vi "Launch Endpoint Actor.vi"(8 "error in (no error)":errorcluster, 11 "Test in":refnum<class "Test.lvclass">) -> (0 "error out":errorcluster, 3 "Test out":refnum<class "Test.lvclass">)   [LabVIEW 2019, in "Test.lvlib" / "Test.lvclass"]
uses:
  Test.lvclass
  C:/Program Files (x86)/National Instruments/LabVIEW 2019/vi.lib/ActorFramework/Actor/Actor.lvclass
  <vilib>/NI/Actors/Network Endpoint Actors/Nested Endpoint/Nested Endpoint/Nested Endpoint.lvclass
  C:/Program Files (x86)/National Instruments/LabVIEW 2019/vi.lib/NI/Actors/Network Endpoint Actors/Network Endpoint/Network Endpoint/Network Endpoint.lvclass
  Test Messages/Endpoint Connected Msg/Endpoint Connected Msg.lvclass
  C:/Program Files (x86)/National Instruments/LabVIEW 2019/vi.lib/NI/Actors/Network Endpoint Actors/Nested Endpoint/Nested Endpoint Messages/Connected Msg/Connected Msg.lvclass
  Test.lvclass/Test.ctl
  <vilib>/NI/Actors/Network Endpoint Actors/Network Endpoint/Network Endpoint/Network Endpoint.lvclass/Network Endpoint.ctl
  <vilib>/NI/Actors/Network Endpoint Actors/Nested Endpoint/Nested Endpoint/Nested Endpoint.lvclass/Nested Endpoint.ctl
  <vilib>/NI/Actors/Network Endpoint Actors/Network Endpoint/Network Endpoint/Network Endpoint.lvclass
  <vilib>/ActorFramework/Actor/Actor.lvclass
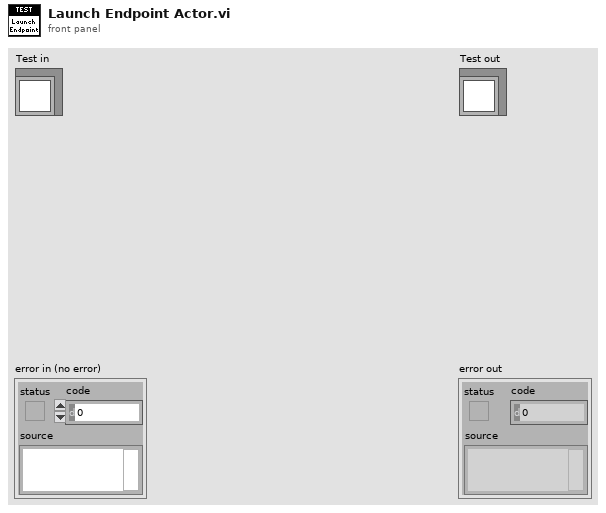
[diagram p1: front panel]
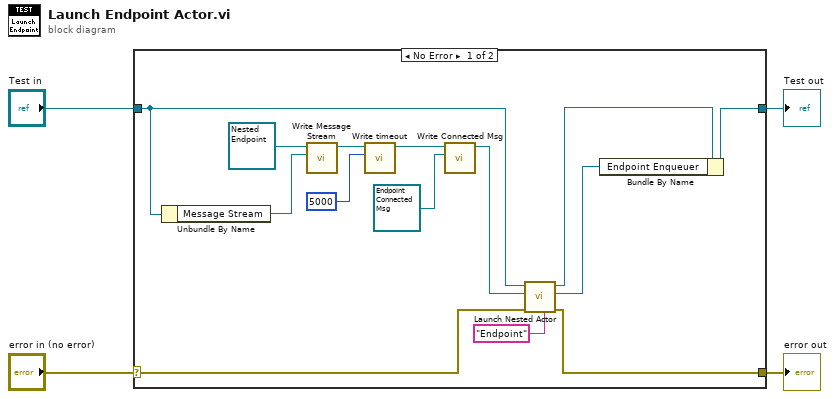
[diagram p0: block diagram]
diagram:
  n1 = case shown="No Error" "error in (no error)" {
    selector: "error in (no error)" -> [w10 w20]
    tunnel: [w9 w20] -> w3
    tunnel: [w6 w19] -> w1
    tunnel: "Test in" -> [w8 w19]
    frame No Error {
      n2 = Unbundle By Name(w8) -> ("Message Stream"=w17:refnum<class "Message Stream.lvclass">)
      n3 = call <vilib>:"Write Message Stream.vi"("Message Stream"=w17, "Network Endpoint in"=refnum<class "Nested Endpoint.lvclass"> refnum ("Nested Endpoint.lvlib:Nested Endpoint.lvclass")) -> ("Network Endpoint out"=w14:refnum<class "Nested Endpoint.lvclass">)  [unwired: 9 in]
      n4 = call <vilib>:"Write timeout.vi"("timeout"=5000, "Network Endpoint in"=w14) -> ("Network Endpoint out"=w15:refnum<class "Nested Endpoint.lvclass">)  [unwired: 9 in]
      n5 = call <vilib>:"Write Connected Msg.vi"("Nested Endpoint.lvlib:Connected Msg.lvclass"=refnum<class "Endpoint Connected Msg.lvclass"> refnum ("Test.lvlib:Endpoint Connected Msg.lvclass"), "Nested Endpoint in"=w15) -> ("Nested Endpoint out"=w11:refnum<class "Nested Endpoint.lvclass">)  [unwired: 9 in]
      n6 = call <vilib>:"Launch Nested Actor.vi"("Debug Alias"="Endpoint", "error in (no error)"=w10, "Nested Actor"=w11, "Caller Actor in"=w8) -> ("error out"=w9:errorcluster, "Nested Actor's Enqueuer"=w18:refnum<class "Message Enqueuer.lvclass">, "Caller Actor out"=w7:refnum<class "Test.lvclass">)  [unwired: 5 in]
      n7 = Bundle By Name(cluster=w7, "Endpoint Enqueuer"=w18) -> (w6:refnum<class "Test.lvclass">)
    }
    frame Error {
    }
  }
  "error out" <- w3
  "Test out" <- w1
